vi "Copy File to Clipboard.vi"(7 "Picture Ref":refnum<vi>, 8 "error in":errorcluster, 10 "State":string, 11 "File Info":T1) -> (0 "error out":errorcluster)   [LabVIEW 2020, in "Peer Review.lvclass"]
uses:
  Peer Review.lvclass
  TypeDefs/File Info.ctl
  TypeDefs/File State.ctl
  TypeDefs/VI Type.ctl
  <vilib>/Utility/miscctls.llb/LVBoundsTypeDef.ctl
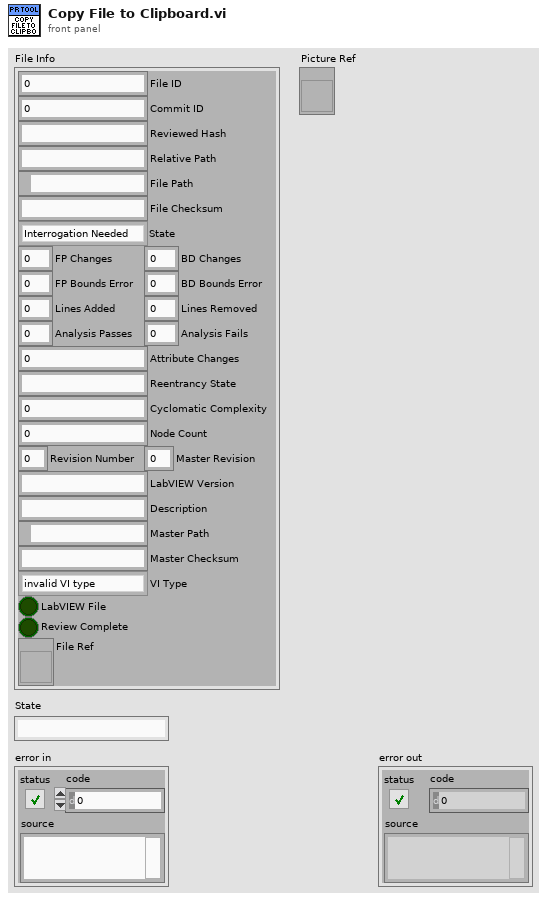
[diagram p1: front panel]
types:
  T1 = typedef "Peer Review.lvclass/File Info.ctl" = cluster{"File ID":i32, "Commit ID":i32, "Reviewed Hash":string, "Relative Path":string, "File Path":path, "File Checksum":string, "State":T2, "FP Changes":i32, "BD Changes":i32, "FP Bounds Error":dbl, "BD Bounds Error":dbl, "Lines Added":i32, "Lines Removed":i32, "Analysis Passes":i32, "Analysis Fails":i32, "Attribute Changes":i32, "Reentrancy State":string, "Cyclomatic Complexity":i32, "Node Count":i32, "Revision Number":u32, "LabVIEW Version":string, "Description":string, "Master Path":path, "Master Checksum":string, "VI Type":T3, "LabVIEW File":bool, "Review Complete":bool, "File Ref":refnum<vi>, "Master Revision":u32}
  T2 = typedef "Peer Review.lvclass/File State.ctl" = enum16{"Interrogation Needed", "Modified", "Deleted", "Added", "Matches Previous", "No Changes", "Moved", "Empty File"}
  T3 = typedef "Peer Review.lvclass/VI Type.ctl" = enum32{"invalid VI type", "Standard VI", "Control VI", "Global VI", "Polymorphic VI", "Configuration VI", "SubSystem", "Facade VI", "Method VI", "Statechart Diagram VI"}
  T4 = cluster{"Font Name:":string, "Size":i16, "Strikeout?":bool, "Italic?":bool, "Underline?":bool, "Outline?":bool, "Shadow?":bool, "Bold?":bool}
  T5 = typedef "LVBoundsTypeDef.ctl" = cluster{"Width":u32, "Height":u32}
  T6 = typedef "imagedata.ctl" = cluster{"image type":i32, "image depth":i32, "image":u8[], "mask":u8[], "colors":u32[], "Rectangle":cluster{"left":i16, "top":i16, "right":i16, "bottom":i16}}
  T7 = cluster{"left":i16, "top":i16, "right":i16, "bottom":i16}
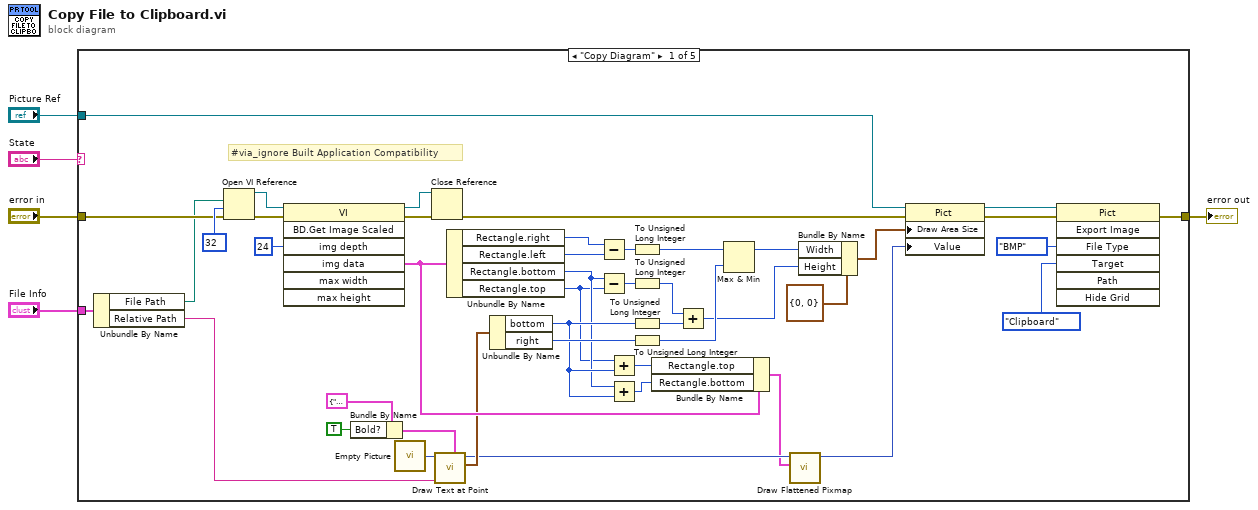
[diagram p0: block diagram]
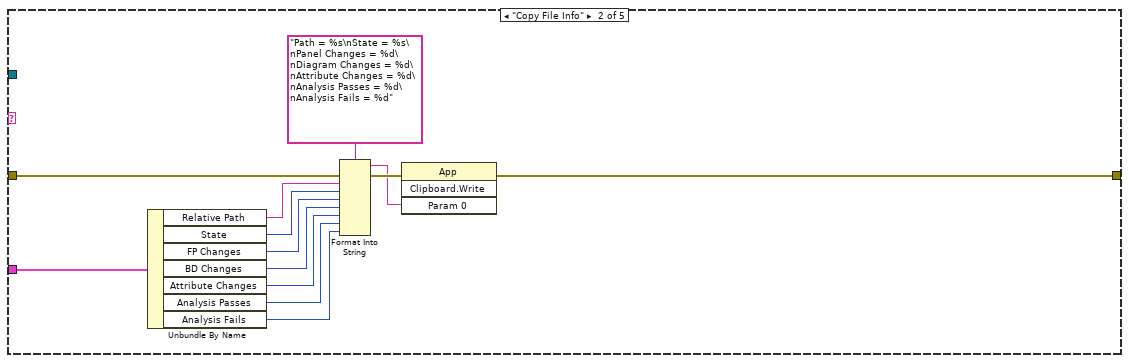
[diagram p2: hidden frame]
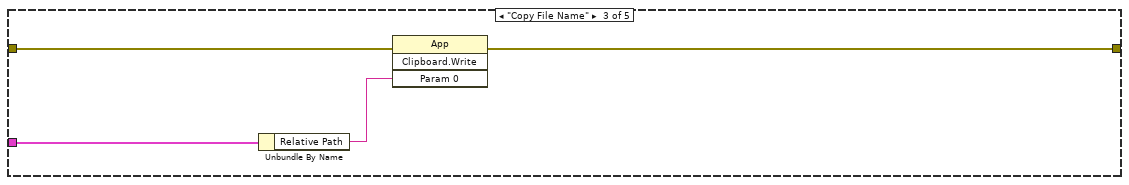
[diagram p3: hidden frame]
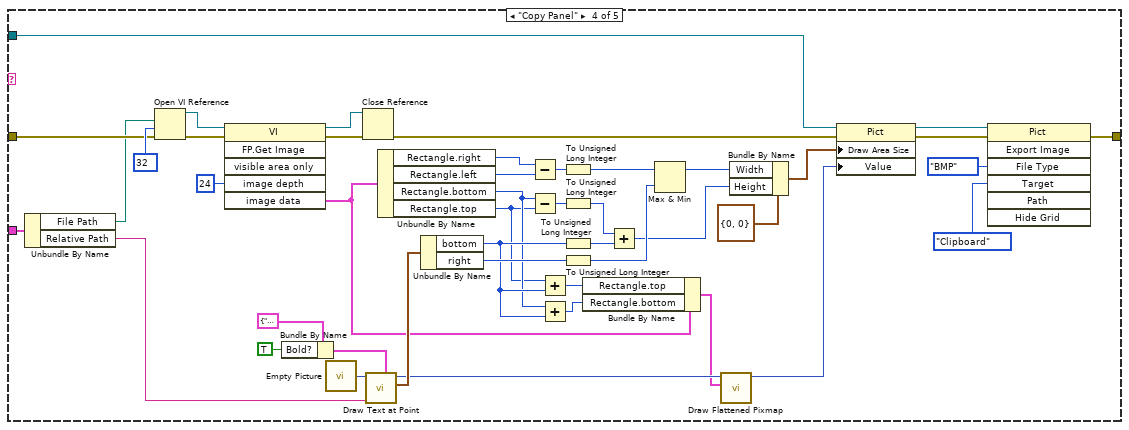
[diagram p4: hidden frame]
diagram:
  n1 = case shown="\"Copy Diagram\"" "State" {
    tunnel: "File Info" -> [w49 w62 w66 w110 _]
    tunnel: [w46 w61 w65 w107 w111] -> w4
    tunnel: "error in" -> [w13 w60 w63 w76 w111]
    tunnel: "Picture Ref" -> [w12 _ _ w75 _]
    frame "Copy Diagram" {
      # "#via_ignore Built Application Compatibility"
      n2 = Unbundle By Name(w49) -> ("File Path"=w11:path, "Relative Path"=w10:string)
      n3 = Open VI Reference(vi path=w11, options=32, error in (no error)=w13) -> (vi reference=w20:refnum<vi>, error out=w19:errorcluster)  [unwired: 3 in]
      n4 = invoke on="Invoke Node" class="VI" method="BD.Get Image Scaled"(reference=w20, error in=w19, "img depth"=24 ("Image Depth")) -> (reference out=w22:refnum<vi>, error out=w21:errorcluster, "img data"=w45:T6)  [unwired: 4 in, 4 out]
      n5 = Bundle By Name(cluster=T4 {"Font Name:"="", "Size"=12, "Strikeout?"=FALSE, "Italic?"=FALSE, "Underline?"=FALSE, "Outline?"=FALSE, "Shadow?"=FALSE, "Bold?"=FALSE} ("[user-specified font]"), "Bold?"=TRUE) -> (w7:T4)
      n6 = call "Empty Picture"() -> ("empty picture"=w9:picture)
      n7 = Close Reference(reference=w22, error in (no error)=w21) -> (error out=w23:errorcluster)
      n8 = call <vilib>:"Draw Text at Point.vi"("[user-specified font]"=w7, "text"=w10, "picture"=w9) -> ("text rect"=w38:T7, "new picture"=w36:picture)  [unwired: 7 in]
      n9 = Unbundle By Name(w45) -> ("Rectangle.right"=w24:i16, "Rectangle.left"=w25:i16, "Rectangle.bottom"=w33:i16, "Rectangle.top"=w31:i16)
      n10 = Unbundle By Name(w38) -> ("bottom"=w39:i16, "right"=w40:i16)
      n11 = Subtract(x=w24, y=w25) -> (x-y=w26:i16)
      n12 = Subtract(x=w33, y=w31) -> (x-y=w27:i16)
      n13 = Add(x=w31, y=w39) -> (x+y=w32:i16)
      n14 = Add(x=w33, y=w39) -> (x+y=w34:i16)
      n15 = To Unsigned Long Integer(number=w26) -> (unsigned 32bit integer=w41:u32)
      n16 = To Unsigned Long Integer(number=w27) -> (unsigned 32bit integer=w29:u32)
      n17 = To Unsigned Long Integer(number=w39) -> (unsigned 32bit integer=w43:u32)
      n18 = To Unsigned Long Integer(number=w40) -> (unsigned 32bit integer=w44:u32)
      n19 = Bundle By Name(cluster=w45, "Rectangle.top"=w32, "Rectangle.bottom"=w34) -> (w35:T6)
      n20 = Add(x=w29, y=w43) -> (x+y=w30:u32)
      n21 = Max & Min(x=w41, y=w44) -> (max(x,y)=w42:u32)  [unwired: 1 out]
      n22 = call <vilib>:"Draw Flattened Pixmap.vi"("image data"=w35, "picture"=w36) -> ("new picture"=w37:picture)  [unwired: 7 in]
      n23 = Bundle By Name(cluster=T5 {"Width"=0, "Height"=0} ("Draw Area Size"), "Width"=w42, "Height"=w30) -> (w28:T5)
      n24 = property on="Property Node" class="Pict"(reference=w12, error in=w23, "Draw Area Size"=w28, "Value"=w37) -> (reference out=w14:refnum<vi>, error out=w15:errorcluster)
      n25 = invoke on="Invoke Node" class="Pict" method="Export Image"(reference=w14, error in=w15, "File Type"=enum32{"BMP", "EPS", "EMF", "PICT"}."BMP", "Target"=enum32{"File", "Clipboard"}."Clipboard") -> (error out=w46:errorcluster)  [unwired: 3 in, 6 out]
    }
    frame "Copy File Info" {
      n26 = Unbundle By Name(w62) -> ("Relative Path"=w58:string, "State"=w55:T2, "FP Changes"=w54:i32, "BD Changes"=w53:i32, "Attribute Changes"=w52:i32, "Analysis Passes"=w51:i32, "Analysis Fails"=w50:i32)
      n27 = Format Into String(format string="Path = %s\nState = %s\nPanel Changes = %d\nDiagram Changes = %d\nAttribute Changes = %d\nAnalysis Passes = %d\nAnalysis Fails = %d", error in=w60, w58, w55, w54, w53, w52, w51, w50) -> (resulting string=w57:string, error out=w59:errorcluster)  [unwired: 1 in]
      n28 = invoke on="Invoke Node" class="App" method="Clipboard.Write"(error in=w59, "Param 0"=w57) -> (error out=w61:errorcluster)  [unwired: 2 in, 3 out]
    }
    frame "Copy File Name" {
      n29 = Unbundle By Name(w66) -> ("Relative Path"=w64:string)
      n30 = invoke on="Invoke Node" class="App" method="Clipboard.Write"(error in=w63, "Param 0"=w64) -> (error out=w65:errorcluster)  [unwired: 2 in, 3 out]
    }
    frame "Copy Panel" {
      n31 = Unbundle By Name(w110) -> ("File Path"=w74:path, "Relative Path"=w73:string)
      n32 = Open VI Reference(vi path=w74, options=32, error in (no error)=w76) -> (vi reference=w82:refnum<vi>, error out=w81:errorcluster)  [unwired: 3 in]
      n33 = invoke on="Invoke Node" class="VI" method="FP.Get Image"(reference=w82, error in=w81, "image depth"=24 ("Image Depth")) -> (reference out=w84:refnum<vi>, error out=w83:errorcluster, "image data"=w67:T6)  [unwired: 3 in, 3 out]
      n34 = Bundle By Name(cluster=T4 {"Font Name:"="", "Size"=12, "Strikeout?"=FALSE, "Italic?"=FALSE, "Underline?"=FALSE, "Outline?"=FALSE, "Shadow?"=FALSE, "Bold?"=FALSE} ("[user-specified font]"), "Bold?"=TRUE) -> (w70:T4)
      n35 = call "Empty Picture"() -> ("empty picture"=w72:picture)
      n36 = Close Reference(reference=w84, error in (no error)=w83) -> (error out=w85:errorcluster)
      n37 = call <vilib>:"Draw Text at Point.vi"("[user-specified font]"=w70, "text"=w73, "picture"=w72) -> ("text rect"=w100:T7, "new picture"=w98:picture)  [unwired: 7 in]
      n38 = Unbundle By Name(w67) -> ("Rectangle.right"=w86:i16, "Rectangle.left"=w87:i16, "Rectangle.bottom"=w95:i16, "Rectangle.top"=w93:i16)
      n39 = Unbundle By Name(w100) -> ("bottom"=w101:i16, "right"=w102:i16)
      n40 = Subtract(x=w86, y=w87) -> (x-y=w88:i16)
      n41 = Subtract(x=w95, y=w93) -> (x-y=w89:i16)
      n42 = Add(x=w93, y=w101) -> (x+y=w94:i16)
      n43 = Add(x=w95, y=w101) -> (x+y=w96:i16)
      n44 = To Unsigned Long Integer(number=w88) -> (unsigned 32bit integer=w103:u32)
      n45 = To Unsigned Long Integer(number=w89) -> (unsigned 32bit integer=w91:u32)
      n46 = To Unsigned Long Integer(number=w101) -> (unsigned 32bit integer=w105:u32)
      n47 = To Unsigned Long Integer(number=w102) -> (unsigned 32bit integer=w106:u32)
      n48 = Bundle By Name(cluster=w67, "Rectangle.top"=w94, "Rectangle.bottom"=w96) -> (w97:T6)
      n49 = Add(x=w91, y=w105) -> (x+y=w92:u32)
      n50 = Max & Min(x=w103, y=w106) -> (max(x,y)=w104:u32)  [unwired: 1 out]
      n51 = call <vilib>:"Draw Flattened Pixmap.vi"("image data"=w97, "picture"=w98) -> ("new picture"=w99:picture)  [unwired: 7 in]
      n52 = Bundle By Name(cluster=T5 {"Width"=0, "Height"=0} ("Draw Area Size"), "Width"=w104, "Height"=w92) -> (w90:T5)
      n53 = property on="Property Node" class="Pict"(reference=w75, error in=w85, "Draw Area Size"=w90, "Value"=w99) -> (reference out=w77:refnum<vi>, error out=w78:errorcluster)
      n54 = invoke on="Invoke Node" class="Pict" method="Export Image"(reference=w77, error in=w78, "File Type"=enum32{"BMP", "EPS", "EMF", "PICT"}."BMP", "Target"=enum32{"File", "Clipboard"}."Clipboard") -> (error out=w107:errorcluster)  [unwired: 3 in, 6 out]
    }
    frame Default {
    }
  }
  "error out" <- w4
